vi "IHS.vi"() -> ()   [LabVIEW 2022 SP3]
doc: "This Labview program is made to run and administere the insect sampling system, using a Universal Robots UR-5 cobot. An Arduino Nano and the developd SRS system."
uses:
  <vilib>/userdefined/High Color/IMAQdx.ctl
  <vilib>/vision/driver/NI_Vision_Acquisition_Software.lvlib
panel:
  in  "Tab Control 2":T1(tab)
  in  "Max. number of insects to try and Pick":dbl=8.0
  in  "Save Pictures":bool=TRUE
  in  "Critical variable":dbl=8.0 format="%#_13g"
  in  "8 Insects or less":bool
  in  "Force botton":bool
  in  "Force command":string="(0,0,0,0,0,0,0,0)"
  out "Listening":bool
  in  "Sample ID":string="Default"
  in  "Training Picture":bool
  in  "Simulate robot connection":bool
  in  "Tip 2 Max insect lengh":dbl=1.5
  in  "Tip 3 Max insect lengh":dbl=3.0
  in  "Tip 4 Max insect lengh":dbl=5.2
  in  "Tip 1 Min insect lengh":dbl=0.3
  in  "Stop Program":bool
  in  "Pause Program":bool
  in  "Start Robot":bool
  in  "Tab Control":enum32{"Communication", "Images", "Data Arrey"}(tab)
  in  "Z, Height":dbl format="%#_13g"
  out "Number of objects in pick-up area":dbl
  out "Insects taken from current picture":dbl
  out "Number of Insects before next picture":dbl
  in  "IP-address":string="192.168.0.10"
  in  "Remote port":u16=30002
  in  "Next Task":string
  out "Message From Robot":string
  out "Object length":dbl
  out "Assignment":string
  out "Corrected Object orientation":dbl
  out "Object CoM Y":dbl
  out "Object CoM X":dbl
  out "Tool":string
  out "Task":string
  in  "Executing Assignment":string
  out "connection ID out":refnum<k5>
  out "XY Graph 3":cluster{dbl[], dbl[]}[](graph)
  out "XY Graph 2":cluster{dbl[], dbl[]}[](graph)
  out "CV Image":T2(plugin-control)
  out "Camera feed":T2(plugin-control)
  out "Insect-data-array":string[][](array[string])
  out "error out":errorcluster
  # "Commands"
  # "Communication to the Robot"
  # "Communication With Robot"
  # "-0.750m<X<0.750m"
  # "Next"
  # "-0.750m<Y<0.750m"
  # "Grapping height [mm]\nBoth tools, keep in limits; +2/-2"
  # "-100°<RZ<100°"
  # "1.0mm<L<25.0mm"
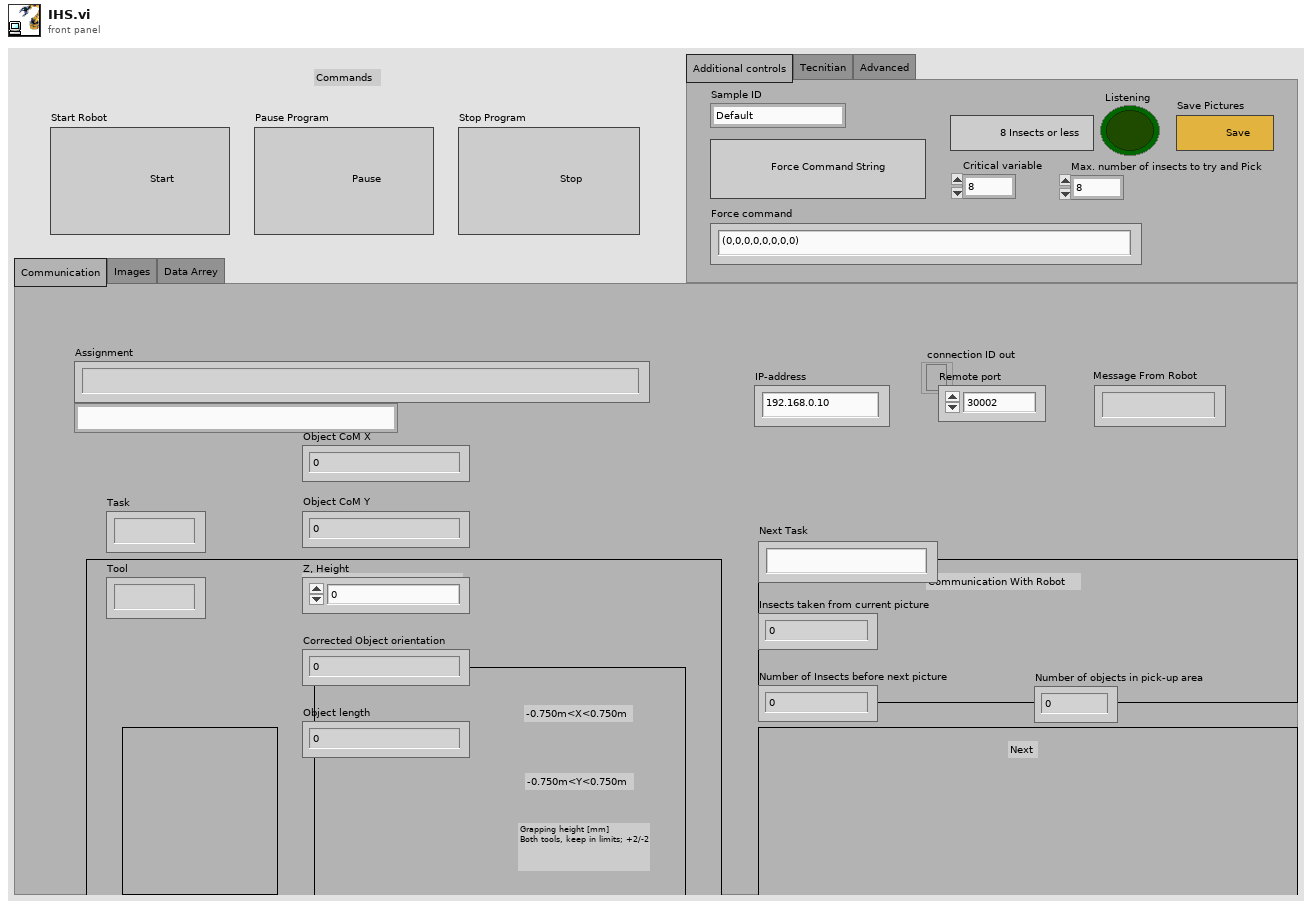
[diagram p1: front panel]
types:
  T1 = enum32{"Additional controls", "Tecnitian", "Advanced"}
  T2 = typedef "IMAQ Image.ctl" = refnum<image>
  T3 = typedef "Image Type" = u32
  T4 = typedef "IMAQdx.ctl" = refnum<k21>
  T5 = cluster{"Image out":T2, "Image Out":T2, "Match Score":i32[], "Number of objects":i32, "Insect-data-array":string[][], bool}
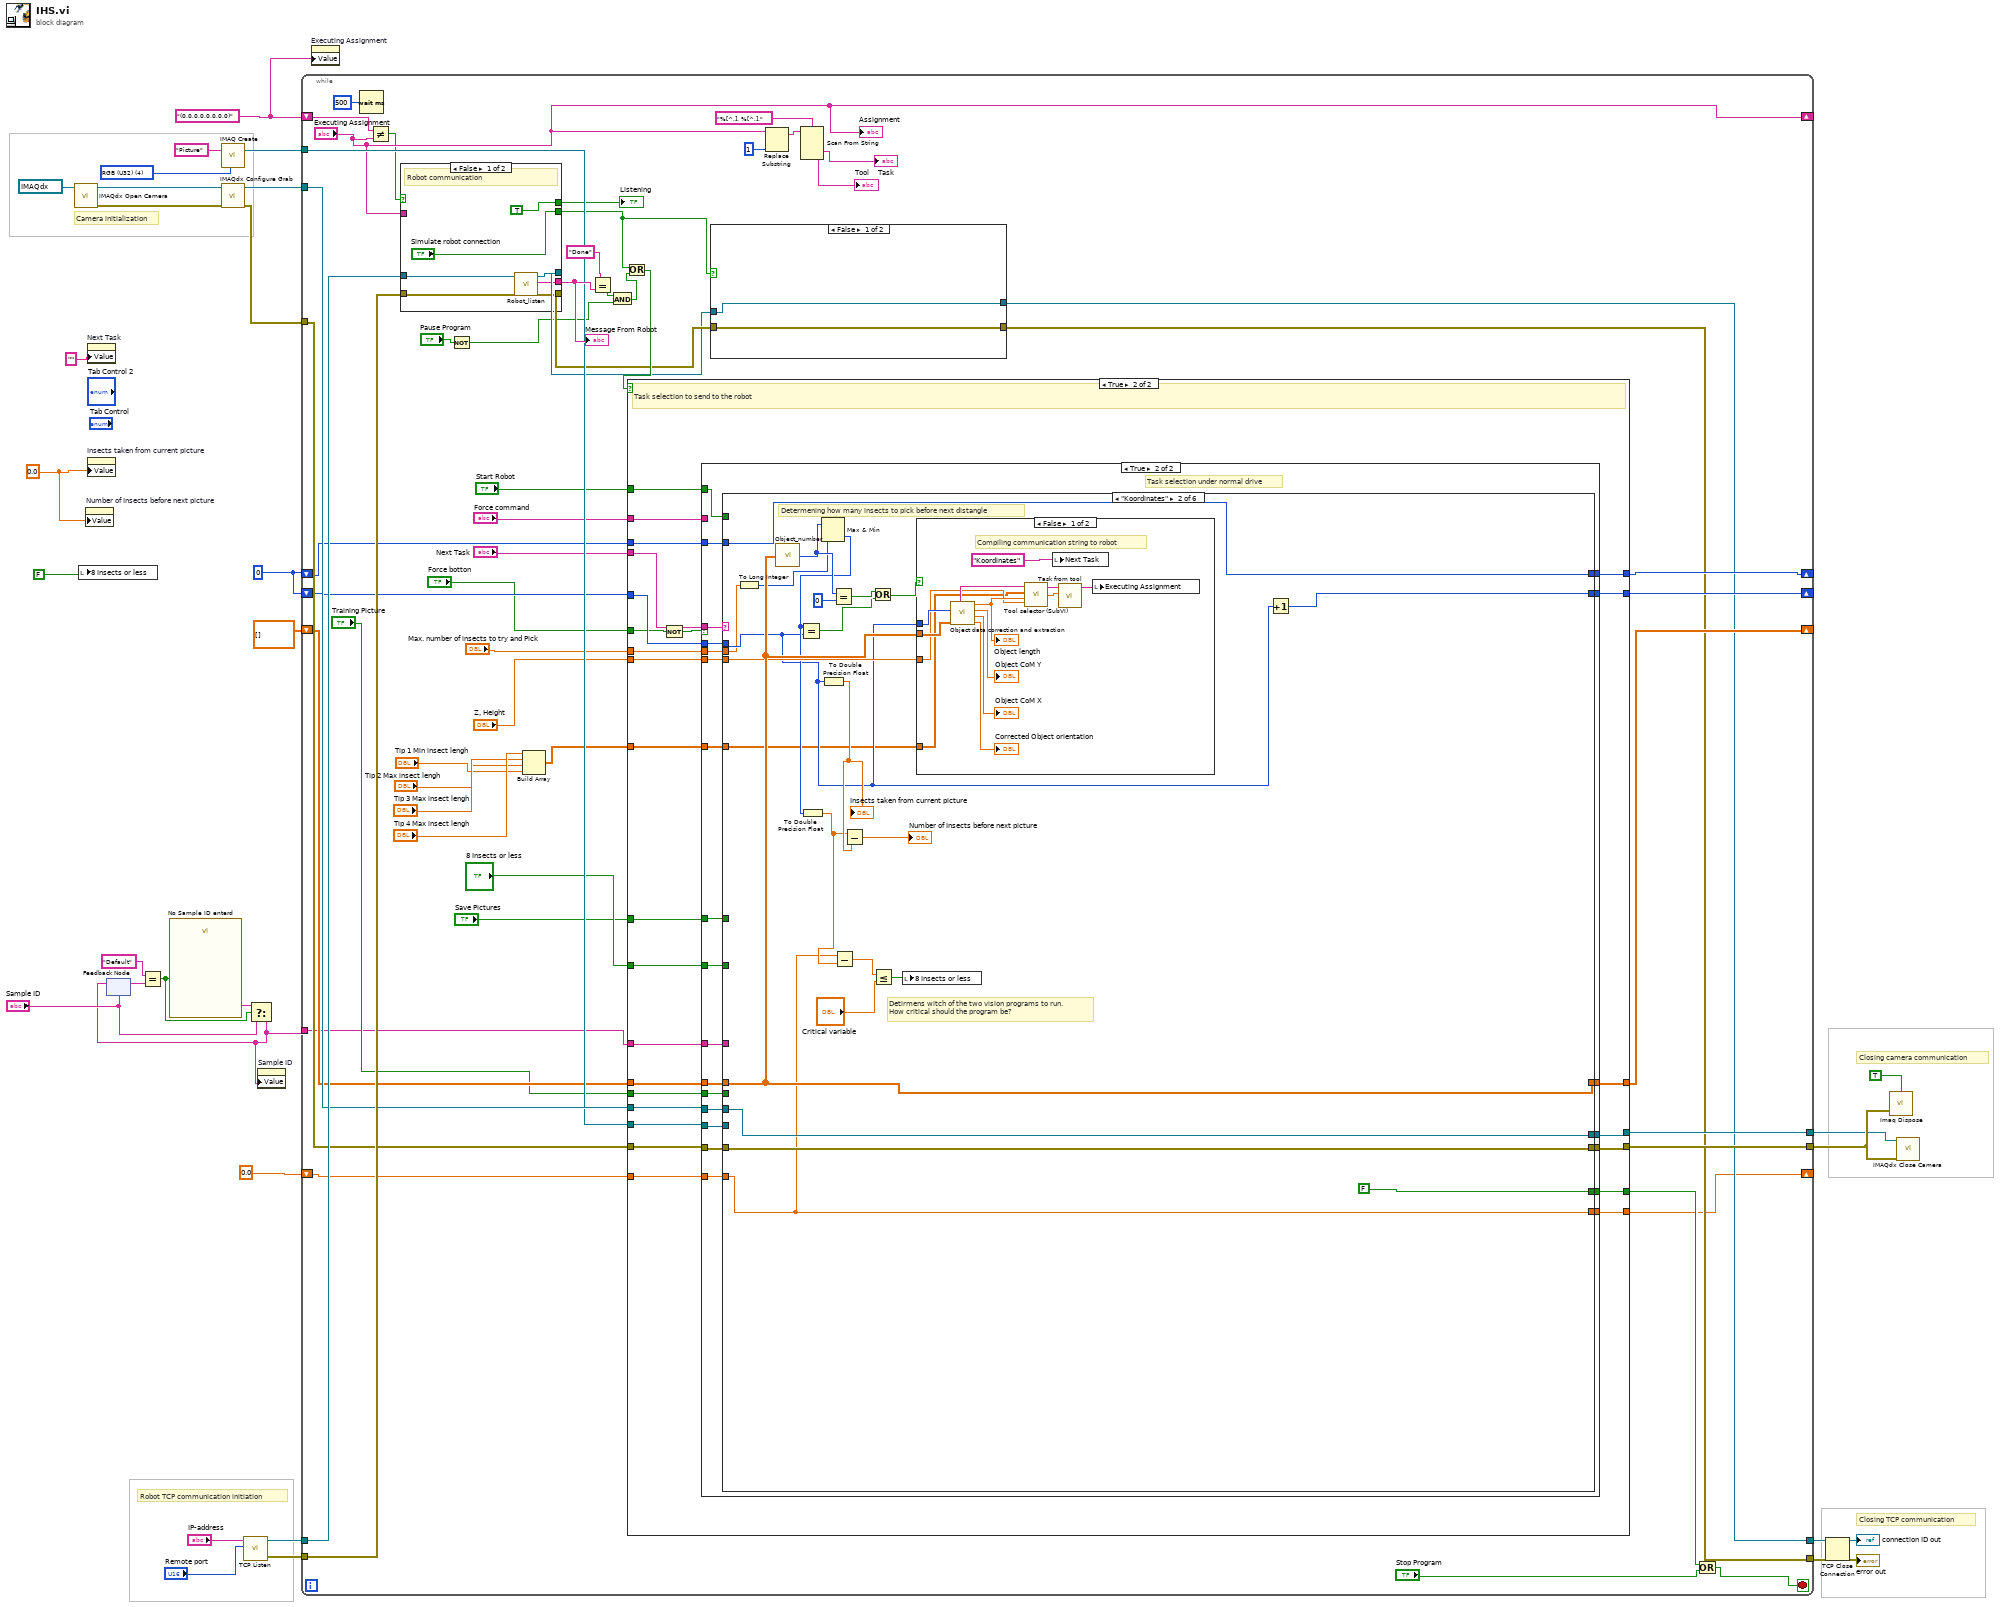
[diagram p0: block diagram]
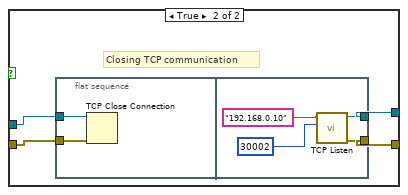
[diagram p2: hidden frame]
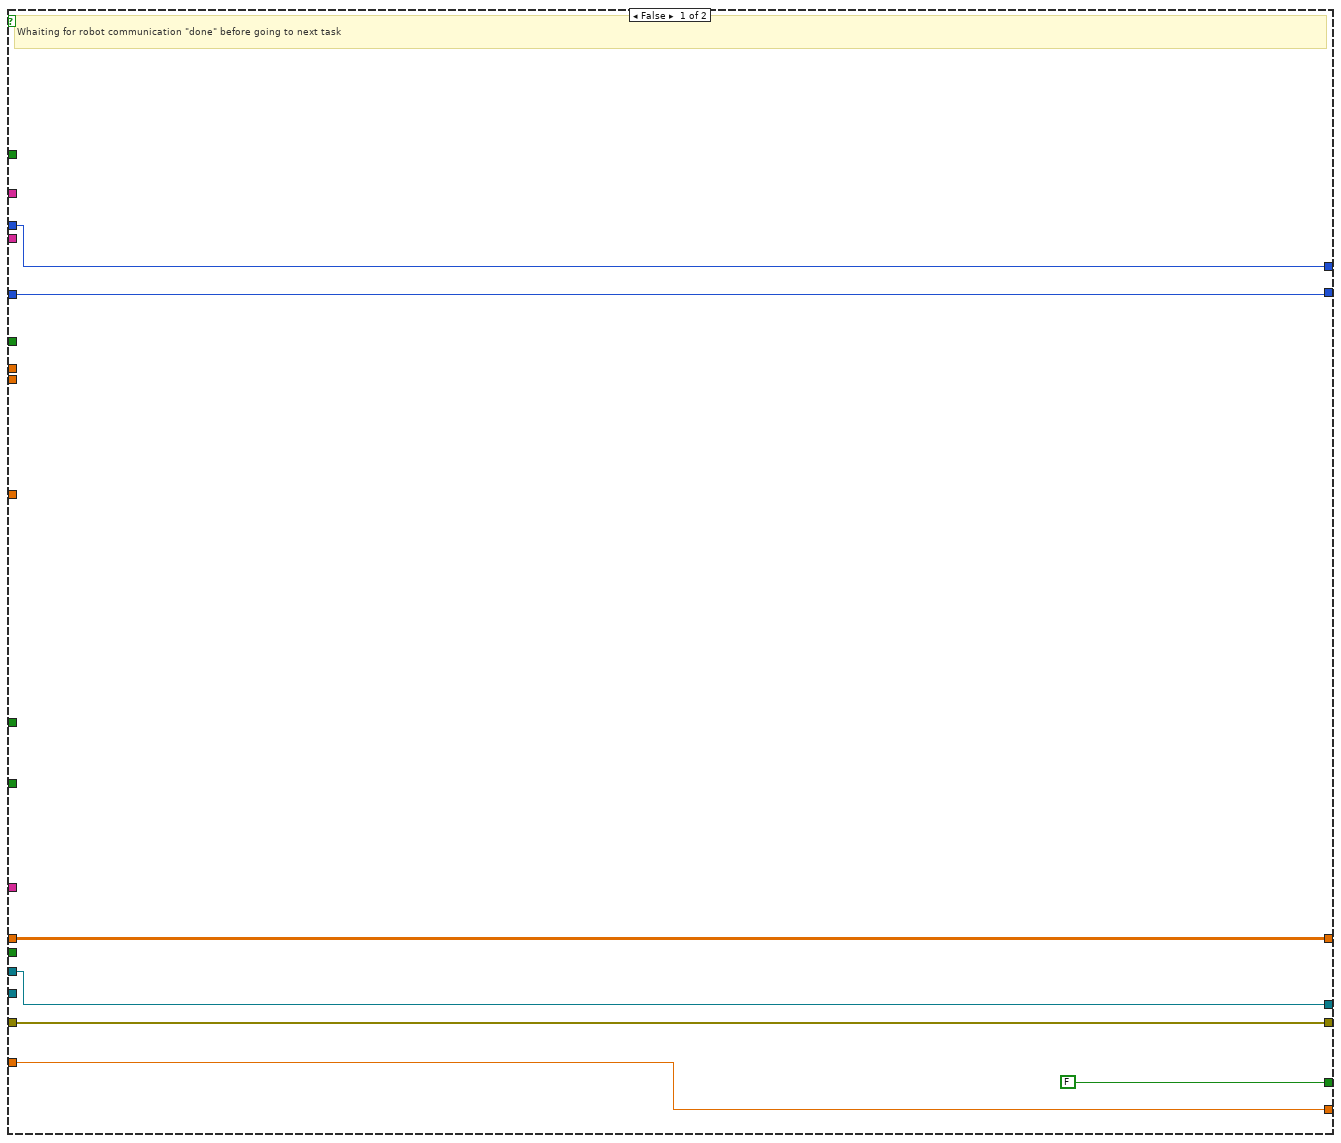
[diagram p3: hidden frame]
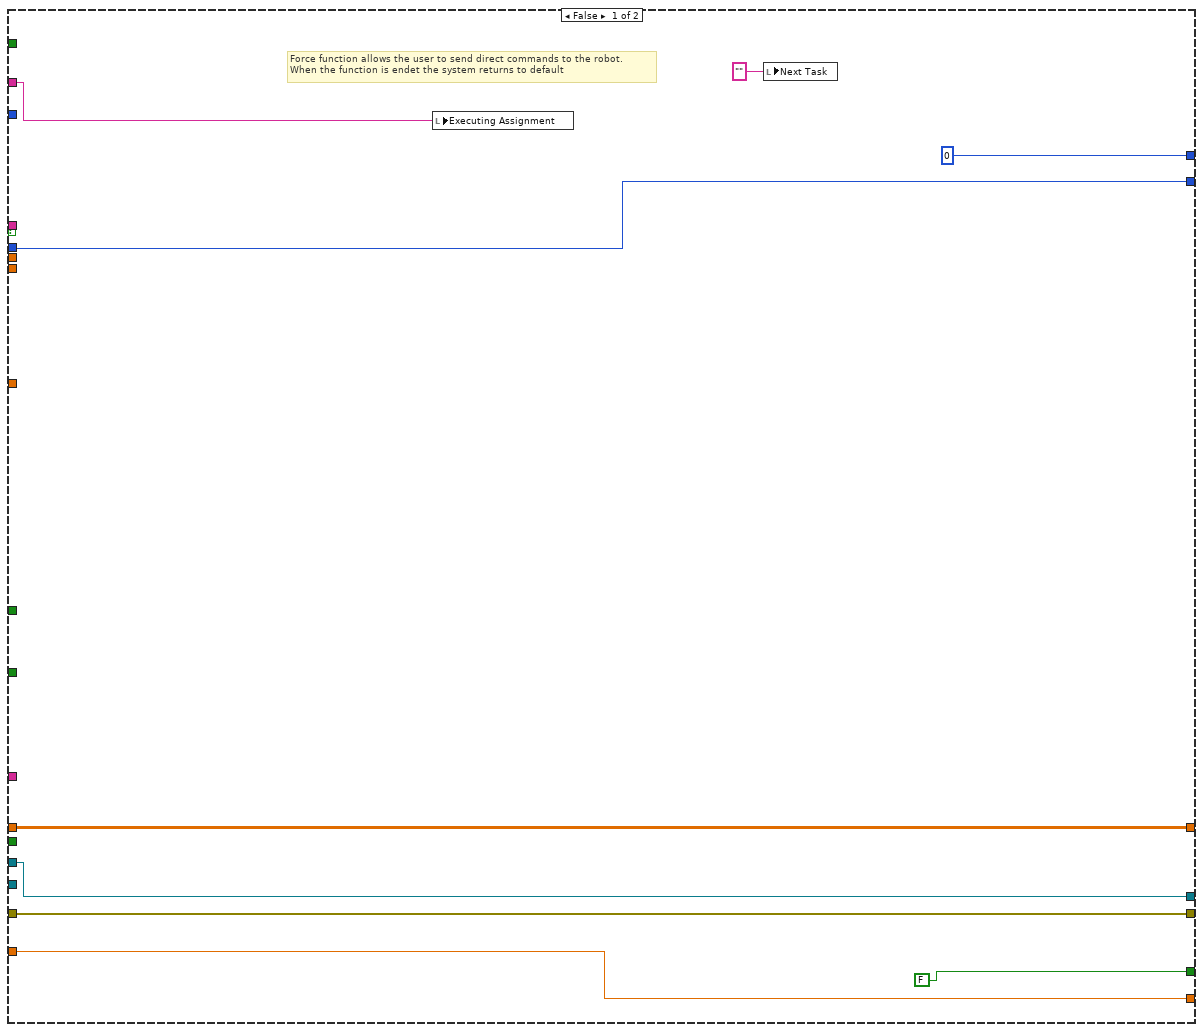
[diagram p4: hidden frame]
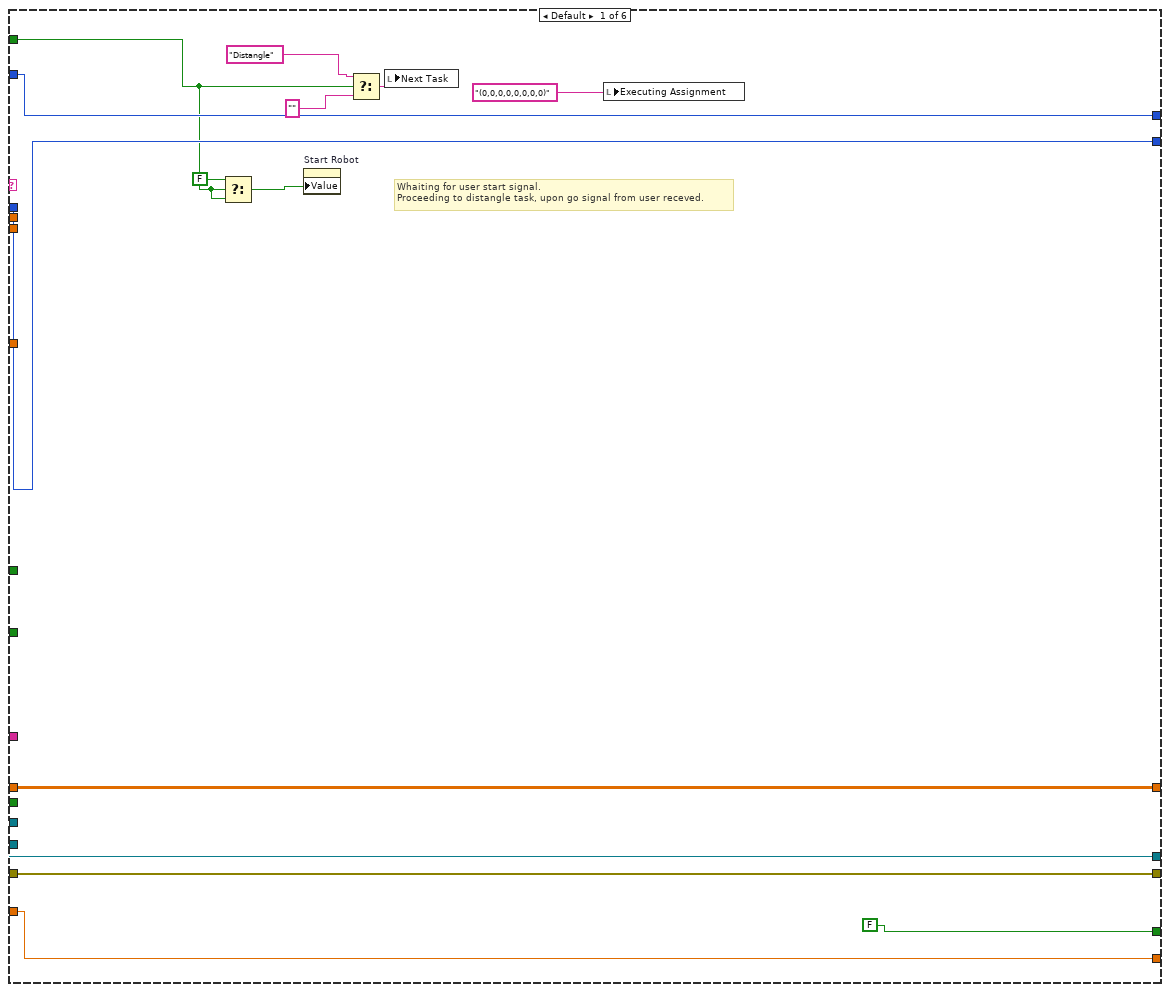
[diagram p5: hidden frame]
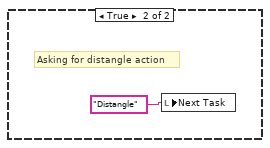
[diagram p6: hidden frame]
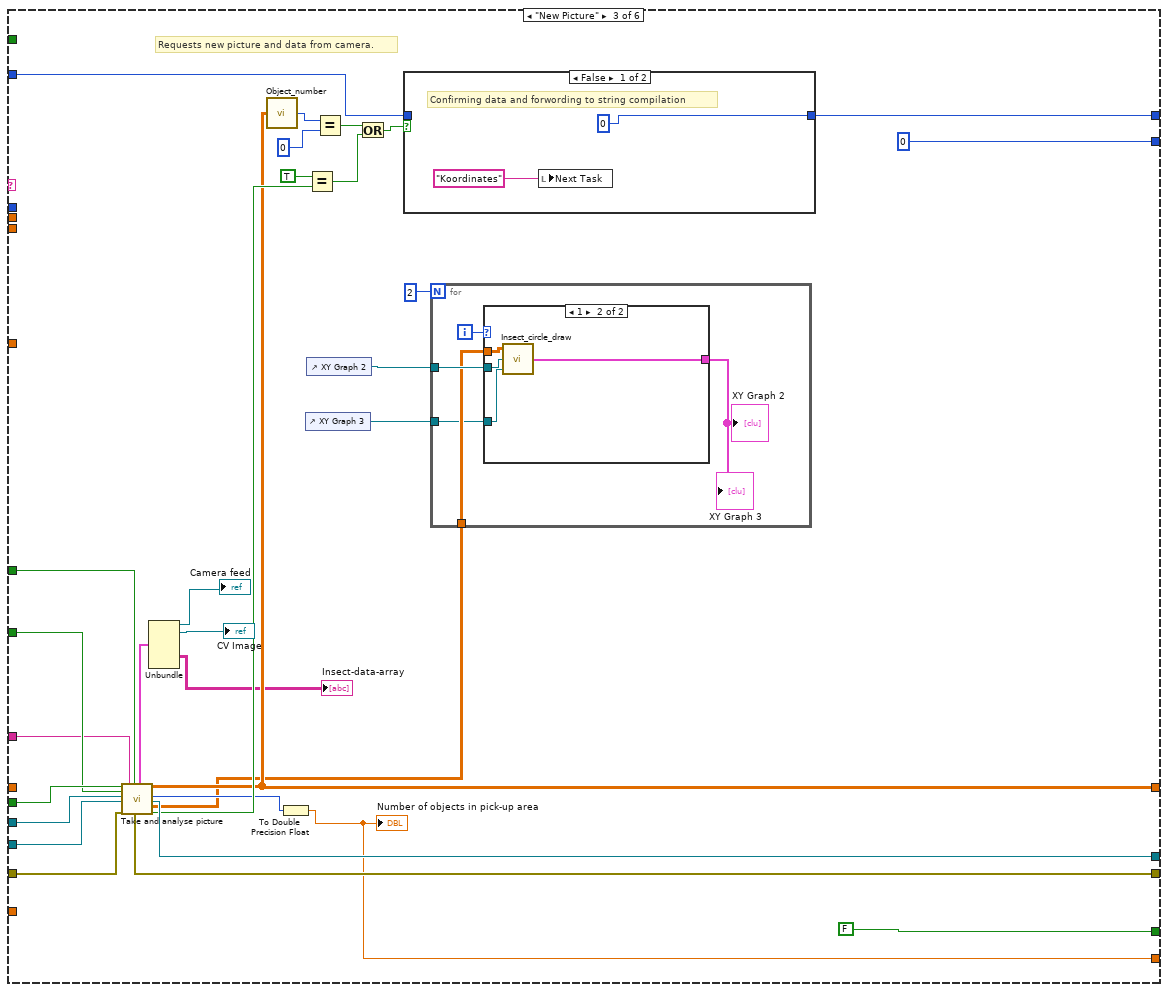
[diagram p7: hidden frame]
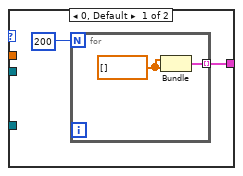
[diagram p8: hidden frame]
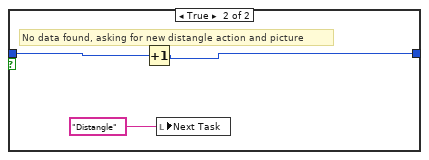
[diagram p9: hidden frame]
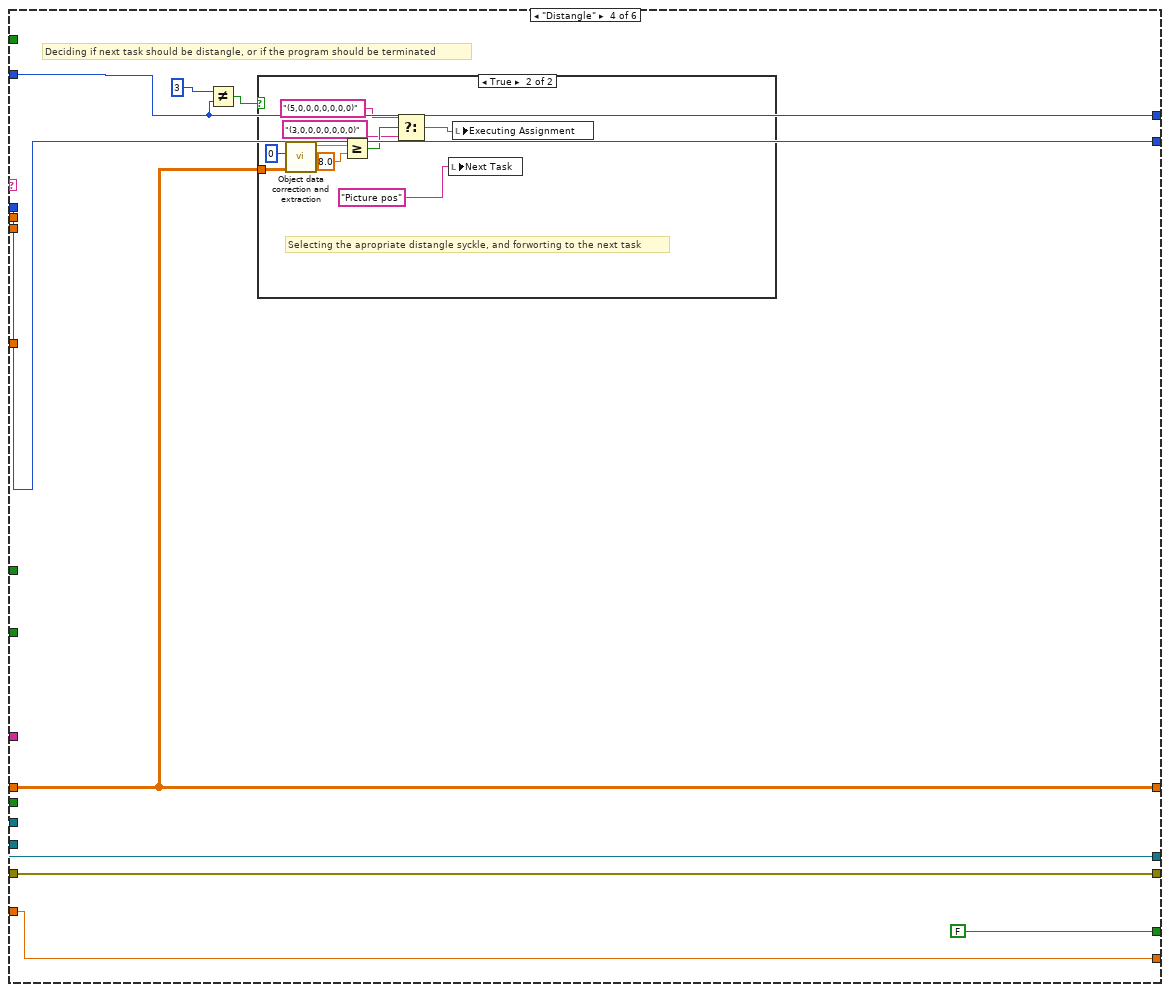
[diagram p10: hidden frame]
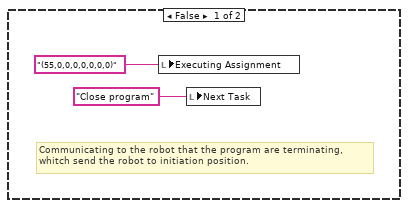
[diagram p11: hidden frame]
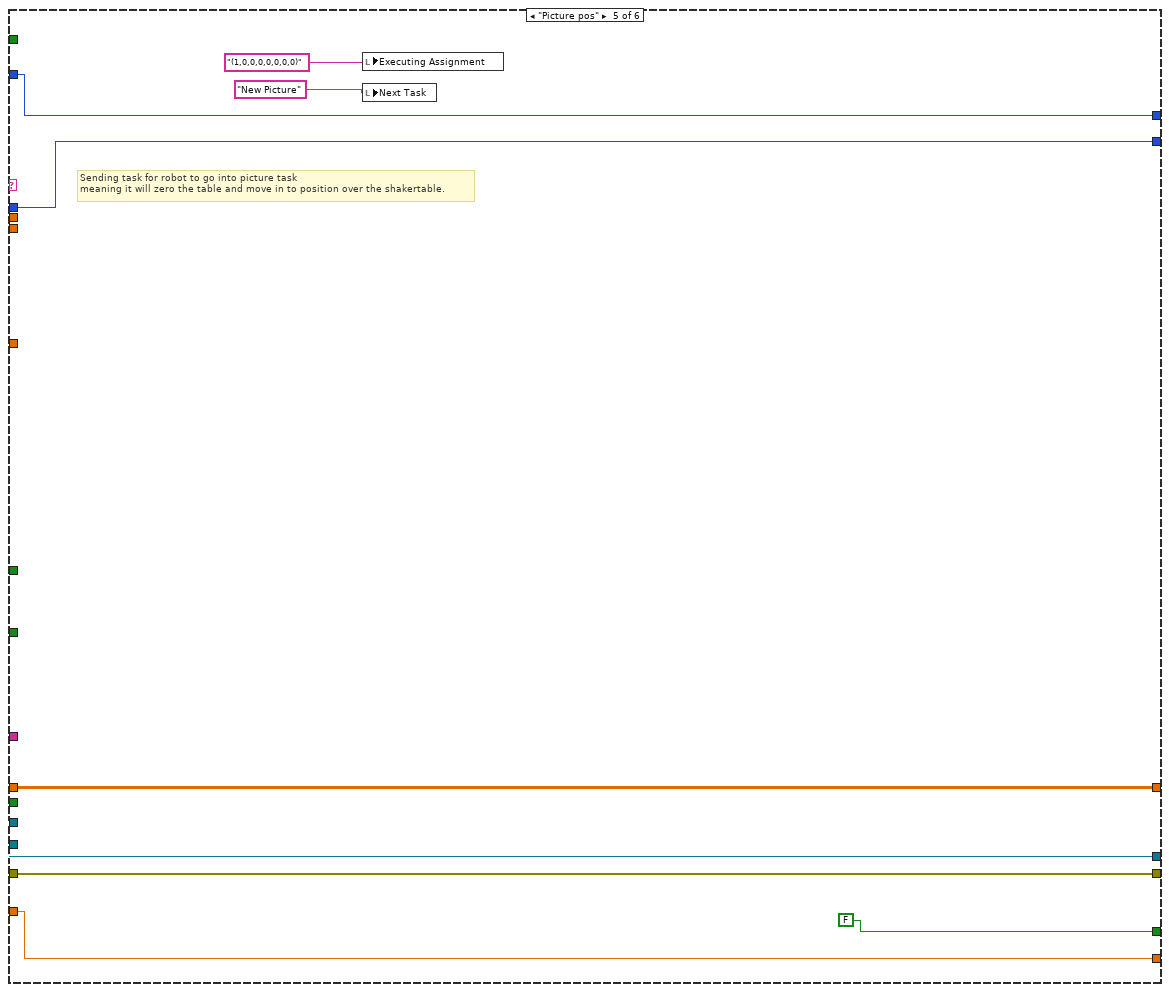
[diagram p12: hidden frame]
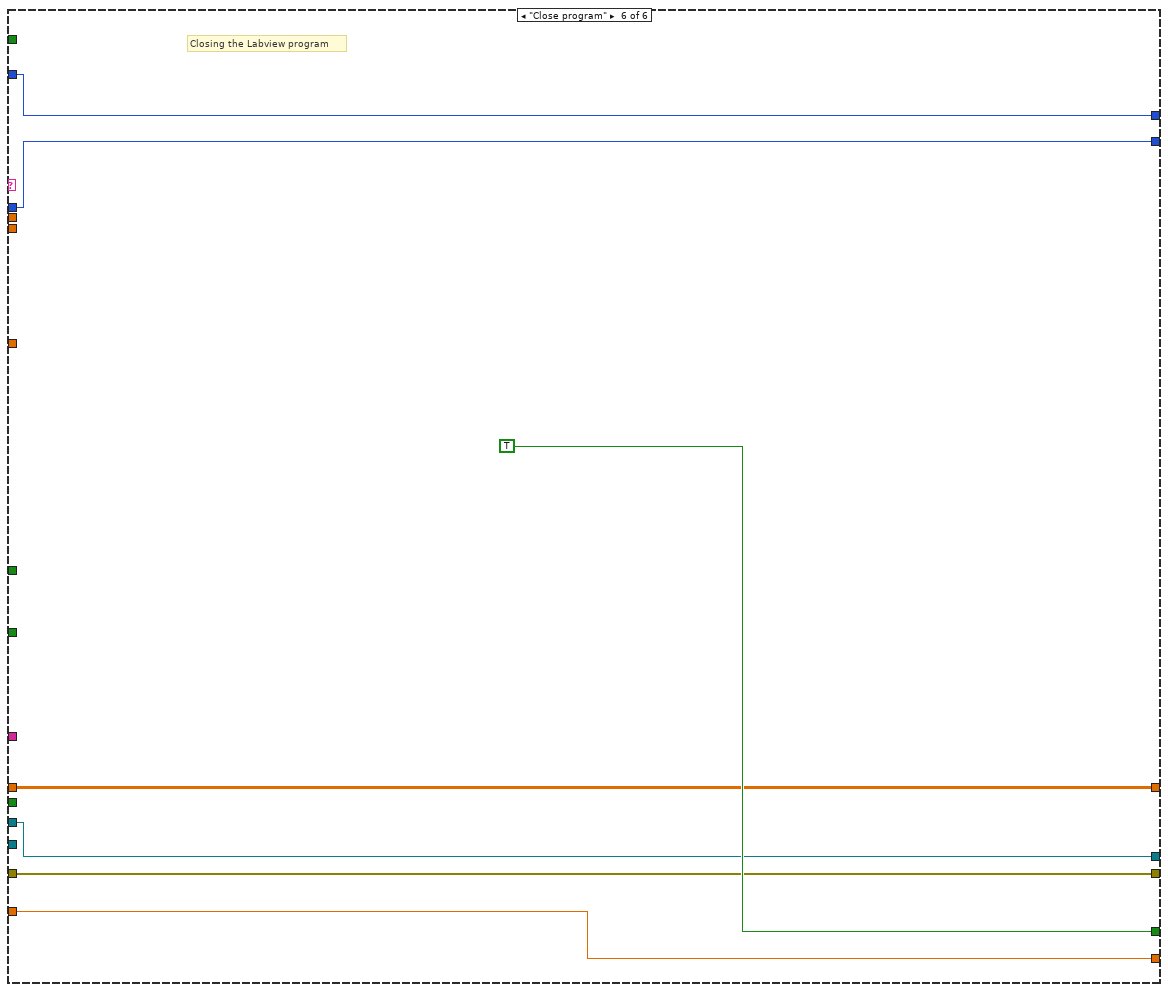
[diagram p13: hidden frame]
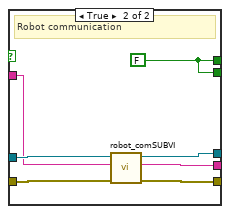
[diagram p14: hidden frame]
diagram:
  w15 = 0.0 ("Insects taken from current picture")
  w18 = 0
  w26 = T3 4 items=["Grayscale (U8)", "Grayscale (I16)", "Grayscale (SGL)", "Complex (CSG)", "RGB (U32)", "HSL (U32)", "RGB (U64)", "Grayscale (U16)"] ("Image Type")
  w17 = "(0,0,0,0,0,0,0,0)"
  # "Closing camera communication"
  # "Closing TCP communication"
  # "Robot TCP communication initiation"
  # "Camera initialization"
  n1 = call <vilib>:"IMAQdx Open Camera.vi"("Session In"=T4 "cam2") -> ("error out"=w27:errorcluster, "Session Out"=w28:T4)  [unwired: 9 in]
  n2 = local write "8 Insects or less"(FALSE ("8 Insects or less")) -> ()
  n3 = property on="Number of Insects before next picture" class="DigNum (strict)"("Value"=w15) -> ()  [unwired: 2 in, 2 out]
  n4 = property on="Next Task" class="Str"("Value"="" ("Task")) -> ()  [unwired: 2 in, 2 out]
  n5 = property on="Insects taken from current picture" class="DigNum (strict)"("Value"=w15) -> ()  [unwired: 2 in, 2 out]
  n6 = feedback #1("Sample ID") -> (w2:string)
  n7 = Equal?(x="Default", y=w2) -> (x = y?=w5:bool)
  n8 = call "No Sample ID enterd"("Enable"=w5) -> ("Sample ID"=w6:string)  [unwired: 16 in, 2 out]
  n9 = call "IMAQ Create"("Image Name"="Picture", "Image Type"=w26) -> ("New Image"=w22:T2)  [unwired: 3 in, 1 out]
  n10 = call <vilib>:"IMAQdx Configure Grab.vi"("error in"=w27, "Session In"=w28) -> ("error out"=w24:errorcluster, "Session Out"=w23:T4)  [unwired: 8 in]
  n11 = call <vilib>:"TCP Listen.vi"("port"="Remote port", "service name"="IP-address") -> ("error out"=w12:errorcluster, "connection ID"=w11:refnum<k5>)  [unwired: 5 in, 3 out]
  n12 = Select(t=w6, s=w5, f="Sample ID") -> (s? t:f=w1:string)
  n13 = feedback-in #1(w1) -> ()
  n14 = property on="Sample ID" class="Str"("Value"=w1) -> ()  [unwired: 2 in, 2 out]
  n15 = while {
    shift-right: ["Executing Assignment"] -> _
    shift-left: w17 -> [w49]
    tunnel: w11 -> [w84]
    tunnel: w12 -> [w83]
    tunnel: w24 -> [w82]
    tunnel: w23 -> [w81]
    tunnel: w22 -> [w80]
    tunnel: [w79] -> w21
    tunnel: [w78] -> w20
    shift-right: [w76] -> _
    shift-left: w18 -> [w74]
    shift-right: [w75] -> _
    shift-left: dbl[][] [] ("Insect-data-array (out of range removed)") -> [w73]
    shift-right: [w71] -> _
    shift-left: w18 -> [w70]
    tunnel: [w51] -> w10
    tunnel: [w50] -> w9
    shift-right: [w43] -> _
    shift-left: 0.0 -> [w42]
    tunnel: w1 -> [w36]
    stop <- w68 stop-if-true
    n16 = Wait (ms)(milliseconds to wait=u32 500) -> ()  [unwired: 1 out]
    n17 = Not Equal?(x=w49, y="Executing Assignment") -> (x != y?=w44:bool)
    n18 = case shown="False" w44 {
      tunnel: w83 -> [w306 w315]
      tunnel: w84 -> [w305 w314]
      tunnel: [w307 w313] -> w53
      tunnel: [w308 w312] -> w52
      tunnel: "Executing Assignment" -> [_ w309]
      tunnel: [w304 w311] -> w85
      tunnel: [TRUE w310] -> w56
      tunnel: ["Simulate robot connection" w310] -> w54
      frame False {
        # "Robot communication"
        n19 = call "Robot_listen.vi"("error in (no error)"=w306, "connection ID IN"=w305) -> ("error IO"=w307:errorcluster, "robotmessage"=w304:string, "connection ID OUT"=w308:refnum<k5>)  [unwired: 7 in]
      }
      frame True {
        w310 = FALSE
        # "Robot communication"
        n20 = call "robot_comSUBVI.vi"("error in (no error)"=w315, "message"=w309, "ConnectionID In"=w314) -> ("error IO"=w313:errorcluster, "robotmessage"=w311:string, "connection ID"=w312:refnum<k5>)  [unwired: 6 in]
      }
    }
    "Message From Robot" <- w85
    "Listening" <- w56
    n21 = Not(x="Pause Program") -> (.not. x?=w45:bool)
    n22 = Build Array("Tip 4 Max insect lengh", "Tip 3 Max insect lengh", "Tip 2 Max insect lengh", "Tip 1 Min insect lengh") -> (w41:dbl[])
    n23 = Equal?(x="Done", y=w85) -> (x = y?=w47:bool)
    n24 = And(x=w47, y=w45) -> (x .and. y?=w46:bool)
    n25 = Or(x=w54, y=w46) -> (x .or. y?=w55:bool)
    n26 = case shown="True" w55 {
      tunnel: w82 -> [w105 w129]
      tunnel: w81 -> [w106 w131]
      tunnel: w80 -> [_ w130]
      tunnel: [w105 w128] -> w79
      tunnel: [w106 w127] -> w78
      tunnel: w74 -> [w104 w132]
      tunnel: "Training Picture" -> [_ w126]
      tunnel: "Next Task" -> [_ w125]
      tunnel: [w104 w124] -> w76
      tunnel: [w103 w123] -> w75
      tunnel: w73 -> [w103 w122]
      tunnel: "Force botton" -> [_ w117]
      tunnel: "Force command" -> [_ w121]
      tunnel: [w102 w120] -> w71
      tunnel: w70 -> [w102 w119]
      tunnel: "Start Robot" -> [_ w116]
      tunnel: [FALSE w115] -> w67
      tunnel: "Z, Height" -> [_ w114]
      tunnel: "8 Insects or less" -> [_ w113]
      tunnel: [w100 w112] -> w43
      tunnel: w42 -> [w100 w111]
      tunnel: w41 -> [_ w110]
      tunnel: w36 -> [_ w109]
      tunnel: "Save Pictures" -> [_ w108]
      tunnel: "Max. number of insects to try and Pick" -> [_ w107]
      frame False {
        # "Whaiting for robot communication \"done\" before going to next task"
      }
      frame True {
        # "Task selection to send to the robot"
        n27 = Not(x=w117) -> (.not. x?=w118:bool)
        n28 = case shown="True" w118 {
          tunnel: w132 -> [w134 w164]
          tunnel: w131 -> [w140 w163]
          tunnel: w130 -> [_ w162]
          tunnel: w129 -> [w139 w161]
          tunnel: [w139 w160] -> w128
          tunnel: [w140 w159] -> w127
          tunnel: w126 -> [_ w158]
          tunnel: w125 -> [_ w157]
          tunnel: [w134 w156] -> w124
          tunnel: [w141 w155] -> w123
          tunnel: w122 -> [w141 w154]
          tunnel: w121 -> [w135 _]
          tunnel: [0 w153] -> w120
          tunnel: w119 -> [_ w152]
          tunnel: w116 -> [_ w151]
          tunnel: [FALSE w150] -> w115
          tunnel: w114 -> [_ w149]
          tunnel: w113 -> [_ w148]
          tunnel: [w133 w147] -> w112
          tunnel: w111 -> [w133 w146]
          tunnel: w110 -> [_ w145]
          tunnel: w109 -> [_ w144]
          tunnel: w108 -> [_ w143]
          tunnel: w107 -> [_ w142]
          frame False {
            # "Force function allows the user to send direct commands to the robot.\nWhen the function is endet the system returns to default"
            n29 = local write "Executing Assignment"(w135) -> ()
            n30 = local write "Next Task"("" ("Next Task")) -> ()
          }
          frame True {
            # "Task selection under normal drive"
            n31 = case shown="\"Koordinates\"" w157 {
              tunnel: w158 -> [_ _ w247 _ _ _]
              tunnel: w164 -> [w178 w187 _ w274 w287 w299]
              tunnel: w163 -> [w176 w188 w246 w273 w291 w297]
              tunnel: w162 -> [_ _ w245 _ _ _]
              tunnel: w161 -> [w175 w202 w244 w272 w292 w296]
              tunnel: [w175 w202 w243 w272 w292 w296] -> w160
              tunnel: [w176 w188 w242 w273 w291 w297] -> w159
              tunnel: [w178 w192 0 w274 w287 w299] -> w156
              tunnel: [w177 w201 w239 w267 w293 w298] -> w155
              tunnel: w154 -> [w177 w201 _ w267 w293 w298]
              tunnel: [w174 w198 w232 w271 w289 w300] -> w153
              tunnel: w152 -> [w174 w198 w231 w271 w289 w300]
              tunnel: w151 -> [w168 _ _ _ _ _]
              tunnel: [FALSE FALSE FALSE FALSE FALSE TRUE] -> w150
              tunnel: w149 -> [_ w191 _ _ _ _]
              tunnel: w148 -> [_ _ w219 _ _ _]
              tunnel: [w165 w182 w220 w266 w286 w295] -> w147
              tunnel: w146 -> [w165 w182 _ w266 w286 w295]
              tunnel: w145 -> [_ w181 _ _ _ _]
              tunnel: w144 -> [_ _ w218 _ _ _]
              tunnel: w143 -> [_ _ w217 _ _ _]
              tunnel: w142 -> [_ w180 _ _ _ _]
              frame Default {
                # "Whaiting for user start signal.\nProceeding to distangle task, upon go signal from user receved."
                n32 = Select(t=FALSE, s=w168, f=w168) -> (s? t:f=w169:bool)
                n33 = property on="Start Robot" class="Bool (strict)"("Value"=w169) -> ()  [unwired: 2 in, 2 out]
                n34 = Select(t="Distangle" ("Task"), s=w168, f="") -> (s? t:f=w172:string)
                n35 = local write "Next Task"(w172) -> ()
                n36 = local write "Executing Assignment"("(0,0,0,0,0,0,0,0)") -> ()
              }
              frame "Koordinates" {
                # "Detirmens witch of the two vision programs to run.\nHow critical should the program be?"
                # "Determening how many insects to pick before next distangle"
                n37 = To Long Integer(number=w180) -> (32bit integer=w179:i32)
                n38 = call "Object_number.vi"("Insect-data-array"=w201) -> ("Number of objects"=w200:i32)
                n39 = Max & Min(x=w200, y=w179) -> (min(x,y)=w189:i32)  [unwired: 1 out]
                n40 = Equal?(x=w189, y=w187) -> (x = y?=w195:bool)
                n41 = To Double Precision Float(number=w189) -> (double precision float=w183:dbl)
                n42 = To Double Precision Float(number=w187) -> (double precision float=w190:dbl)
                "Insects taken from current picture" <- w190
                n43 = Equal?(x=w200, y=0) -> (x = y?=w196:bool)
                n44 = Subtract(x=w182, y=w183) -> (x-y=w184:dbl)
                n45 = Subtract(x=w183, y=w190) -> (x-y=→"Number of Insects before next picture":dbl)
                n46 = Or(x=w196, y=w195) -> (x .or. y?=w197:bool)
                n47 = Less Or Equal?(x=w184, y="Critical variable") -> (x <= y?=w186:bool)
                n48 = local write "8 Insects or less"(w186) -> ()
                n49 = case shown="False" w197 {
                  tunnel: w201 -> [w214 _]
                  tunnel: w187 -> [w213 _]
                  tunnel: w191 -> [w204 _]
                  tunnel: w181 -> [w203 _]
                  frame False {
                    # "Compiling communication string to robot"
                    n50 = call "Object data correction and extraction.vi"("Object-data-array"=w214, "Object number of interest"=w213) -> ("Corrected Object orientation"=→"Corrected Object orientation":dbl, "Object CoM X"=→"Object CoM X":dbl, "Object CoM Y"=→"Object CoM Y":dbl, "Obejct length"=w215:dbl, "Assignment Coordinates"=w210:string)  [unwired: 2 in]
                    "Object length" <- w215
                    n51 = call "Tool selector (SubVI).vi"("Z, Hight"=w204, "Obejct length"=w215, "Tool size values"=w203, "Assignment -Task - Tool"=w210) -> ("Tool"=w212:dbl, "Assignment - Task"=w209:string)  [unwired: 1 out]
                    n52 = local write "Next Task"("Koordinates" ("Task")) -> ()
                    n53 = call "Task from tool.vi"("Tool"=w212, "Assignment - Task"=w209) -> ("Assignment"=w211:string)  [unwired: 8 in, 1 out]
                    n54 = local write "Executing Assignment"(w211) -> ()
                  }
                  frame True {
                    # "Asking for distangle action"
                    n55 = local write "Next Task"("Distangle" ("Task")) -> ()
                  }
                }
                n56 = Increment(x=w187) -> (x+1=w192:i32)
              }
              frame "New Picture" {
                # "Requests new picture and data from camera."
                n57 = call "Take and analyse picture.vi"("Training image on/off"=w247, "8 Insects or less"=w219, "Session Out in"=w246, "Refnum in"=w245, "error in (no error)"=w244, "Sample ID"=w218, "Safe pictures"=w217) -> ("error out"=w243:errorcluster, "output cluster"=w225:T5, "Insect-data-array (out of range removed)"=w239:dbl[][], "Number of objects"=w227:i32, "Session Out out"=w242:T4, "Tegne cirkel array"=w223:dbl[][], "Black image error"=w240:bool)  [unwired: 6 in]
                n58 = Unbundle(w225) -> ("Image out"=→"Camera feed":T2, "Image Out"=→"CV Image":T2, "Insect-data-array"=→"Insect-data-array":string[][])  [unwired: 3 out]
                n59 = call "Object_number.vi"("Insect-data-array"=w239) -> ("Number of objects"=w238:i32)
                n60 = To Double Precision Float(number=w227) -> (double precision float=w220:dbl)
                "Number of objects in pick-up area" <- w220
                n61 = control-ref of="XY Graph 3"() -> (w221:refnum<vi>)
                n62 = Equal?(x=TRUE, y=w240) -> (x = y?=w233:bool)
                n63 = control-ref of="XY Graph 2"() -> (w222:refnum<vi>)
                n64 = Equal?(x=w238, y=0) -> (x = y?=w235:bool)
                n65 = Or(x=w235, y=w233) -> (x .or. y?=w234:bool)
                n66 = case shown="False" w234 {
                  tunnel: [0 w264] -> w232
                  tunnel: w231 -> [_ w263]
                  frame False {
                    # "Confirming data and forwording to string compilation"
                    n67 = local write "Next Task"("Koordinates" ("Task")) -> ()
                  }
                  frame True {
                    # "No data found, asking for new distangle action and picture"
                    n68 = Increment(x=w263) -> (x+1=w264:i32)
                    n69 = local write "Next Task"("Distangle" ("Task")) -> ()
                  }
                }
                n70 = for {
                  N: 2 -> [_]
                  tunnel: w222 -> [w252]
                  tunnel: w223 -> [w250]
                  tunnel: w221 -> [w248]
                  i -> [w251]
                  n71 = case shown="1" w251 {
                    tunnel: w252 -> [_ w260]
                    tunnel: [w253 w259] -> w249
                    tunnel: w250 -> [_ w258]
                    tunnel: w248 -> [_ w257]
                    frame 0, Default {
                      n72 = for {
                        N: 200 -> [_]
                        tunnel: [w256] -> w253 mode=indexing
                        w255 = dbl[] []
                        n73 = Bundle(w255, w255) -> (w256:cluster{dbl[], dbl[]})  [unwired: 1 in]
                      }
                    }
                    frame 1 {
                      n74 = call "Insect_circle_draw.vi"("XYGraph in 2"=w257, "XYGraph in"=w260, "appended array"=w258) -> ("Array"=w259:cluster{dbl[], dbl[]}[])
                    }
                  }
                  "XY Graph 2" <- w249
                  "XY Graph 3" <- w249
                }
              }
              frame "Distangle" {
                # "Deciding if next task should be distangle, or if the program should be terminated"
                n75 = Not Equal?(x=3, y=w271) -> (x != y?=w269:bool)
                n76 = case shown="True" w269 {
                  tunnel: w267 -> [_ w284]
                  frame False {
                    # "Communicating to the robot that the program are terminating,\nwhitch send the robot to initiation position."
                    n77 = local write "Executing Assignment"("(55,0,0,0,0,0,0,0)" ("Executing Assignment")) -> ()
                    n78 = local write "Next Task"("Close program" ("Next Task")) -> ()
                  }
                  frame True {
                    # "Selecting the apropriate distangle syckle, and forworting to the next task"
                    n79 = call "Object data correction and extraction.vi"("Object-data-array"=w284, "Object number of interest"=0) -> ("Obejct length"=w283:dbl)  [unwired: 2 in, 4 out]
                    n80 = Greater Or Equal?(x=w283, y=8.0) -> (x >= y?=w278:bool)
                    n81 = Select(t="(5,0,0,0,0,0,0,0)" ("Assignment"), s=w278, f="(3,0,0,0,0,0,0,0)") -> (s? t:f=w279:string)
                    n82 = local write "Next Task"("Picture pos" ("Task")) -> ()
                    n83 = local write "Executing Assignment"(w279) -> ()
                  }
                }
              }
              frame "Picture pos" {
                # "Sending task for robot to go into picture task\nmeaning it will zero the table and move in to position over the shakertable."
                n84 = local write "Executing Assignment"("(1,0,0,0,0,0,0,0)" ("Assignment")) -> ()
                n85 = local write "Next Task"("New Picture" ("Task")) -> ()
              }
              frame "Close program" {
                # "Closing the Labview program"
              }
            }
          }
        }
      }
    }
    n86 = case shown="False" w54 {
      tunnel: w52 -> [w89 w92]
      tunnel: w53 -> [w88 w93]
      tunnel: [w89 w91] -> w51
      tunnel: [w88 w90] -> w50
      frame False {
      }
      frame True {
        # "Closing TCP communication"
        n87 = flat-sequence {
          tunnel: w93 -> [w95]
          tunnel: w92 -> [w94]
          tunnel: [w97] -> w91
          tunnel: [w96] -> w90
          frame #0 {
            n88 = TCP Close Connection(connection ID=w94, error in (no error)=w95) -> ()  [unwired: 1 in, 2 out]
          }
          frame #1 {
            n89 = call <vilib>:"TCP Listen.vi"("port"=u16 30002 ("Remote port 2"), "service name"="192.168.0.10" ("IP-address 2")) -> ("error out"=w96:errorcluster, "connection ID"=w97:refnum<k5>)  [unwired: 5 in, 3 out]
          }
        }
      }
    }
    n90 = Replace Substring(2:1 ("length (len. of substring)"), 5:"Executing Assignment") -> (1:w60:string)  [unwired: 2 in, 1 out]
    n91 = Scan From String(format string="%[^,], %[^,],", input string=w60) -> (output 1=→"Task":string, output 2=→"Tool":string)  [unwired: 4 in, 3 out]
    n92 = Or(x=w67, y="Stop Program") -> (x .or. y?=w68:bool)
    "Assignment" <- "Executing Assignment"
  }
  n93 = property on="Executing Assignment" class="Str"("Value"=w17) -> ()  [unwired: 2 in, 2 out]
  n94 = TCP Close Connection(connection ID=w10, error in (no error)=w9) -> (connection ID out=→"connection ID out":refnum<k5>, error out=→"error out":errorcluster)  [unwired: 1 in]
  n95 = call "Imaq Dispose"("All Images? (No)"=TRUE, "error in (no error)"=w21) -> ()  [unwired: 4 in, 1 out]
  n96 = call <vilib>:"IMAQdx Close Camera.vi"("error in"=w21, "Session In"=w20) -> ()  [unwired: 9 in, 1 out]
